vi "status.vi"(0 "连接ID":refnum<k5>) -> (1 "连接ID输出":refnum<k5>, 2 "String Value":string)   [LabVIEW 2017]
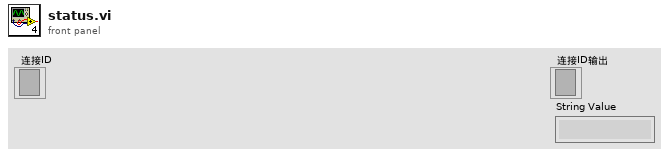
[diagram p1: front panel]
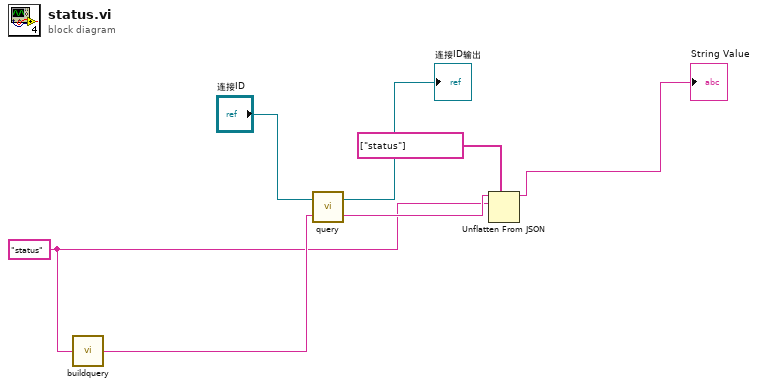
[diagram p0: block diagram]
diagram:
  w3 = "status" ("String")
  n1 = call "buildquery.vi"("String"=w3) -> ("JSON字符串"=w5:string)
  n2 = call "query.vi"("数据输入"=w5, "连接ID"="连接ID") -> ("数据输出"=w4:string, "连接ID输出"=→"连接ID输出":refnum<k5>)
  n3 = Unflatten From JSON(path=string[] ["status"] ("路径"), JSON string=w4, type and defaults=w3) -> (value=→"String Value":string)  [unwired: 4 in, 1 out]
